vi "Read I2C.vi"(6 "NoBlock (F)":bool, 7 "Address":u8, 8 "error in (no error)":errorcluster, 9 "Len":u8, 10 "Bus":u8, 11 "VISA resource name in":refnum<visa-resource-name>) -> (0 "error out":errorcluster, 1 "Data":string, 3 "VISA resource name":refnum<visa-resource-name>)   [LabVIEW 2020, in "CTI-Visa.lvlib"]
uses:
  CTI-Visa.lvlib
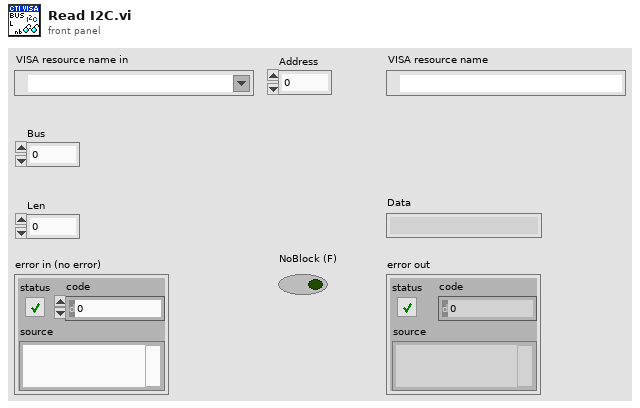
[diagram p1: front panel]
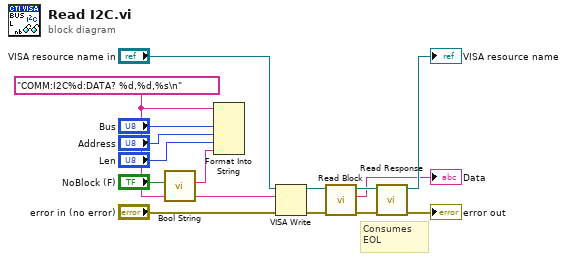
[diagram p0: block diagram]
diagram:
  w11 = "COMM:I2C%d:DATA? %d,%d,%s\n" ("format string")
  # "Consumes EOL"
  n1 = call "Bool String.vi"("Bool"="NoBlock (F)") -> ("String"=w2:string)  [unwired: 10 in]
  n2 = Format Into String(format string=w11, "Bus", "Address", "Len", w2) -> ()  [unwired: 2 in, 2 out]
  n3 = VISA Write(VISA resource name="VISA resource name in", write buffer=w11, error in (no error)="error in (no error)") -> (VISA resource name out=w9:refnum<visa-resource-name>, error out=w10:errorcluster)  [unwired: 1 out]
  n4 = call "Read Block.vi"("error in (no error)"=w10, "VISA resource name in"=w9) -> ("error out"=w8:errorcluster, "Block Data"=→"Data":string, "VISA resource name"=w7:refnum<visa-resource-name>)  [unwired: 7 in]
  n5 = call "Read Response.vi"("error in (no error)"=w8, "VISA resource name in"=w7) -> ("error out"=→"error out":errorcluster, "VISA resource name"=→"VISA resource name":refnum<visa-resource-name>)  [unwired: 7 in, 1 out]
